vi "Write Multi Data Alias.vi"(8 "error in (no error)":errorcluster, 10 "Alias":string, 11 "Multi Data in":refnum<class "Multi Data.lvclass">) -> (0 "error out":errorcluster, 3 "Multi Data out":refnum<class "Multi Data.lvclass">)   [LabVIEW 2020, in "Publisher.lvlib" / "Multi Data.lvclass"]
doc: "Write the Alias to the class."
uses:
  Multi Data.lvclass
  Multi Data.lvclass/Multi Data.ctl
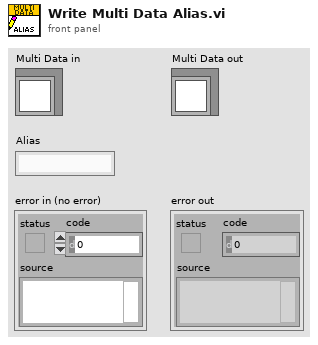
[diagram p1: front panel]
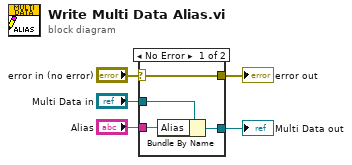
[diagram p0: block diagram]
diagram:
  n1 = case shown="No Error" "error in (no error)" {
    selector: "error in (no error)" -> [w9 w10]
    tunnel: [w9 w10] -> w4
    tunnel: [w7 w11] -> w2
    tunnel: "Multi Data in" -> [w8 w11]
    tunnel: "Alias" -> [w6 _]
    frame No Error {
      n2 = Bundle By Name(cluster=w8, "Alias"=w6) -> (w7:refnum<class "Multi Data.lvclass">)
    }
    frame Error {
    }
  }
  "error out" <- w4
  "Multi Data out" <- w2
